vi "PC_Choose_Best_Shot (DONE).vi"(5 "Table Walls Inputs":sgl[](array[numeric]), 6 "Straight/Bounce":bool, 7 "Puck and Players In":T3, 8 "Error In":errorcluster, 10 "Shot Inputs":cluster{"Bounce":dbl[][], "Straight":dbl[][]}, 11 "Image In":T2) -> (0 "Error Out":errorcluster, 1 "Shot Coordinate":T1, 2 "Best Shot Theta":dbl, 3 "Image Out":T2)   [LabVIEW 2017]
uses:
  <vilib>/vision/Image Controls.llb/IMAQ Image.ctl
panel:
  in  "Wall 1 Angle FF":dbl=4.5 format="%#_13g"
  in  "Wall 3 Angle FF":dbl=2.4 format="%#_13g"
  in  "Shot Coordinate Template":T1
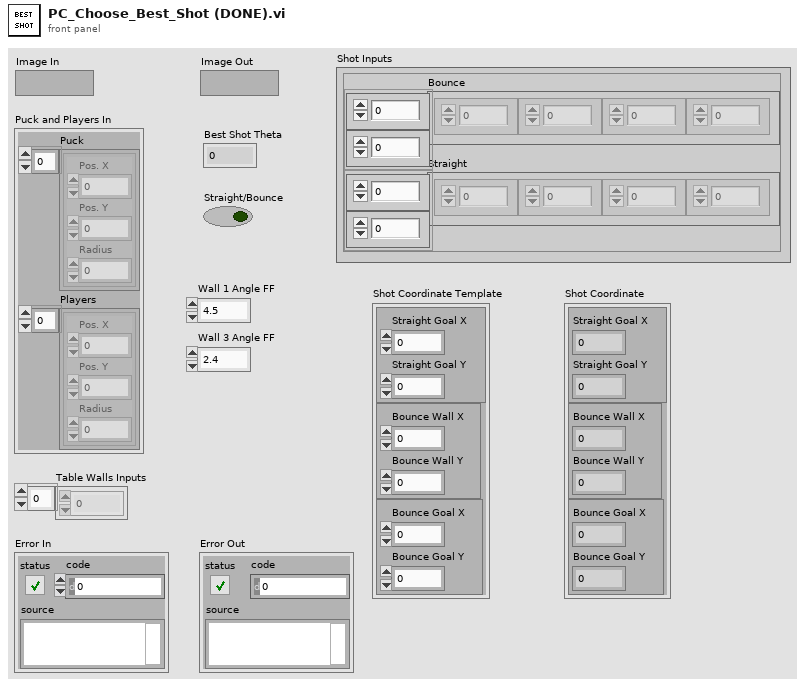
[diagram p1: front panel]
types:
  T1 = cluster{cluster{"Straight Goal X":sgl, "Straight Goal Y":dbl}, cluster{"Bounce Wall X":dbl, "Bounce Wall Y":sgl}, cluster{"Bounce Goal X":sgl, "Bounce Goal Y":dbl}}
  T2 = typedef "IMAQ Image.ctl" = refnum<image>
  T3 = cluster{"Puck":cluster{"Pos. X":i32, "Pos. Y":i32, "Radius":i32}[], "Players":cluster{"Pos. X":i32, "Pos. Y":i32, "Radius":i32}[]}
  T4 = cluster{"Pos. X":i32, "Pos. Y":i32, "Radius":i32}[]
  T5 = cluster{"Pos. X":i32, "Pos. Y":i32, "Radius":i32}
  T6 = cluster{"Numeric Control":sgl, "Numeric Control":dbl}
  T7 = cluster{"Numeric Control":dbl, "Numeric Control":sgl}
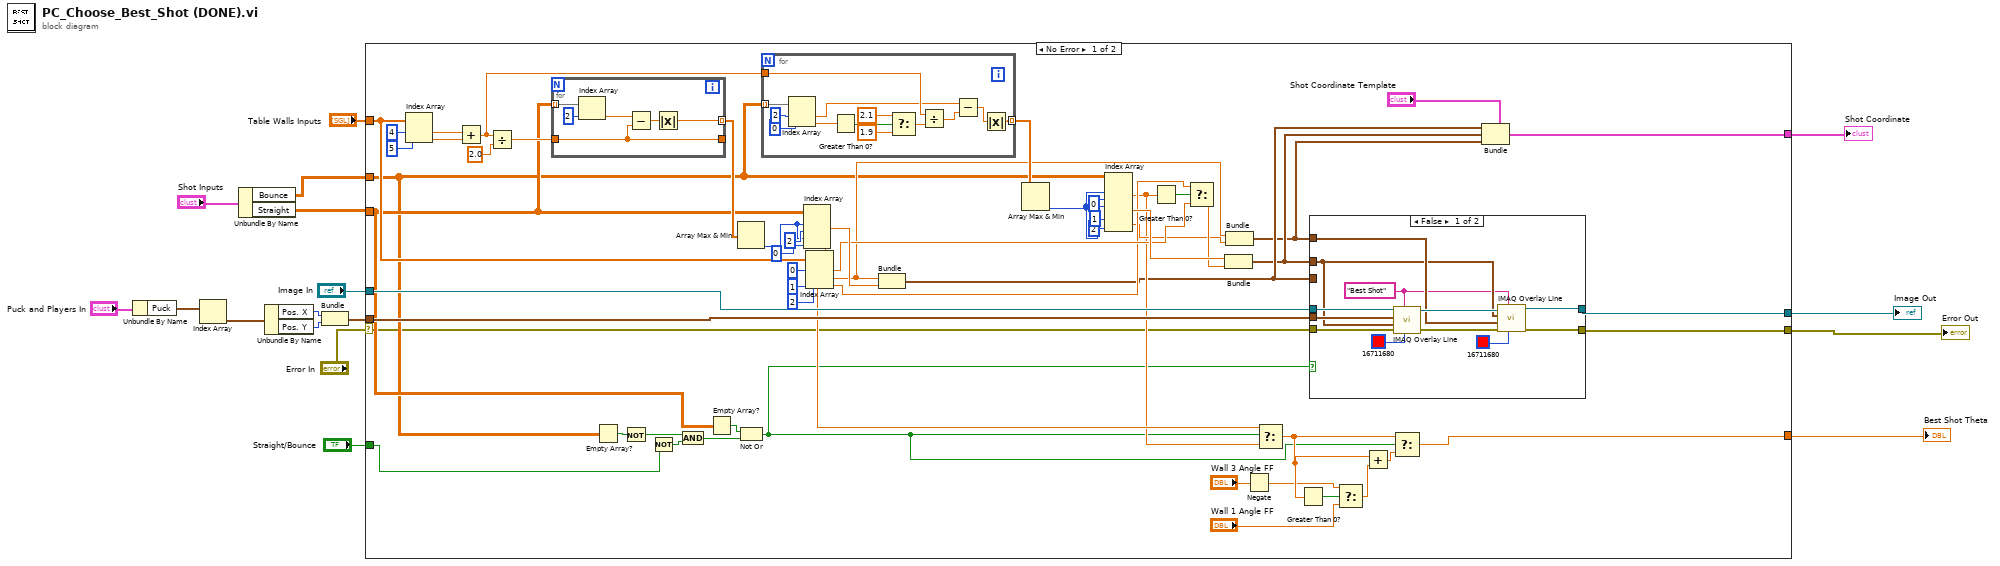
[diagram p0: block diagram]
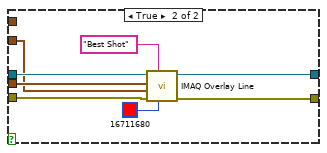
[diagram p2: hidden frame]
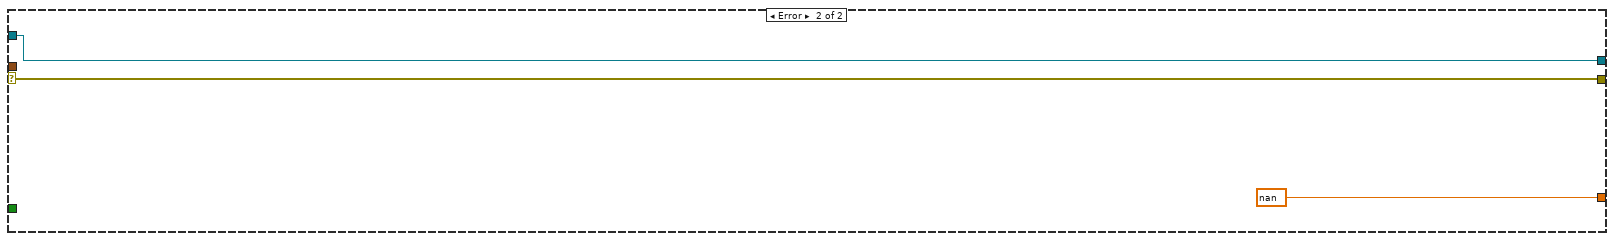
[diagram p3: hidden frame]
diagram:
  n1 = Unbundle By Name("Puck and Players In") -> ("Puck"=w17:T4)
  n2 = Index Array(array=w17) -> (element=w16:T5)  [unwired: 1 in]
  n3 = Unbundle By Name("Shot Inputs") -> ("Bounce"=w3:dbl[][], "Straight"=w2:dbl[][])
  n4 = Unbundle By Name(w16) -> ("Pos. X"=w15:i32, "Pos. Y"=w14:i32)
  n5 = Bundle("Pos. X"=w15, "Pos. Y"=w14) -> (w11:cluster{"Pos. X":i32, "Pos. Y":i32})  [unwired: 1 in]
  n6 = case shown="No Error" "Error In" {
    selector: "Error In" -> [w34 w116]
    tunnel: "Table Walls Inputs" -> [w65 _]
    tunnel: w11 -> [w62 _]
    tunnel: "Image In" -> [w61 w115]
    tunnel: [w60 w116] -> w9
    tunnel: [w59 w115] -> w8
    tunnel: [w27 nan ("Numeric Control")] -> w7
    tunnel: w2 -> [w40 _]
    tunnel: w3 -> [w39 _]
    tunnel: "Straight/Bounce" -> [w28 _]
    tunnel: [w29 _] -> w1
    frame No Error {
      n7 = Index Array(array=w65, index #1=4 ("index"), index #2=5 ("index")) -> (element #1=w72:sgl, element #2=w71:sgl)
      n8 = Add(x=w72, y=w71) -> (x+y=w18:sgl)
      n9 = Divide(x=w18, y=sgl 2.0) -> (x/y=w42:sgl)
      n10 = for {
        tunnel: w40 -> [w113] mode=indexing
        tunnel: w42 -> [w108]
        tunnel: [w109] -> w69 mode=indexing
        tunnel: [w108] -> _
        n11 = Index Array(array=w113, index=2) -> (element=w111:dbl)
        n12 = Subtract(x=w111, y=w108) -> (x-y=w110:dbl)
        n13 = Absolute Value(x=w110) -> (abs(x)=w109:dbl)
      }
      n14 = Empty Array?(array=w39) -> (empty?=w37:bool)
      n15 = Not(x=w37) -> (.not. x?=w36:bool)
      n16 = Not(x=w28) -> (.not. x?=w35:bool)
      n17 = And(x=w36, y=w35) -> (x .and. y?=w41:bool)
      n18 = Empty Array?(array=w40) -> (empty?=w38:bool)
      n19 = Array Max & Min(array=w69) -> (min index (indices)=w46:i32)  [unwired: 3 out]
      n20 = Not Or(1:w41, 2:w38) -> (0:w19:bool)
      n21 = for {
        tunnel: w39 -> [w107] mode=indexing
        tunnel: w18 -> [w98]
        tunnel: [w105] -> w68 mode=indexing
        n22 = Index Array(array=w107, index #1=2 ("index"), index #2=0 ("index")) -> (element #1=w97:dbl, element #2=w103:dbl)
        n23 = Greater Than 0?(x=w103) -> (x > 0?=w102:bool)
        n24 = Select(t=2.1, s=w102, f=1.9) -> (s? t:f=w99:dbl)
        n25 = Divide(x=w98, y=w99) -> (x/y=w96:dbl)
        n26 = Subtract(x=w97, y=w96) -> (x-y=w95:dbl)
        n27 = Absolute Value(x=w95) -> (abs(x)=w105:dbl)
      }
      n28 = Index Array(array=w40, index (row) #1=w46, index (col) #1=2 ("disabled index (col)"), index (row) #2=w46, index (col) #2=0 ("disabled index (col)")) -> (element #1=w63:dbl, element #2=w44:dbl)
      n29 = Index Array(array=w65, index #1=0 ("index"), index #2=1 ("index"), index #3=2 ("index")) -> (element #1=w53:sgl, element #2=w49:sgl, element #3=w50:sgl)
      n30 = Bundle("Numeric Control"=w49, "Numeric Control"=w63) -> (w33:T6)  [unwired: 1 in]
      n31 = Array Max & Min(array=w68) -> (min index (indices)=w47:i32)  [unwired: 3 out]
      n32 = Index Array(array=w39, index (row) #1=w47, index (col) #1=0 ("disabled index (col)"), index (row) #2=w47, index (col) #2=1 ("disabled index (col)"), index (row) #3=w47, index (col) #3=2 ("index (col)")) -> (element #1=w43:dbl, element #2=w56:dbl, element #3=w48:dbl)
      n33 = Greater Than 0?(x=w43) -> (x > 0?=w54:bool)
      n34 = Select(t=w50, s=w54, f=w53) -> (s? t:f=w51:sgl)
      n35 = Bundle("Numeric Control"=w56, "Numeric Control"=w51) -> (w32:T7)  [unwired: 1 in]
      n36 = Bundle("Numeric Control"=w49, "Numeric Control"=w48) -> (w31:T6)  [unwired: 1 in]
      n37 = Negate(x="Wall 3 Angle FF") -> (-x=w22:dbl)
      n38 = Select(t=w44, s=w19, f=w43) -> (s? t:f=w25:dbl)
      n39 = Greater Than 0?(x=w25) -> (x > 0?=w24:bool)
      n40 = case shown="False" w19 {
        tunnel: w34 -> [w84 w93]
        tunnel: w62 -> [w79 w92]
        tunnel: w61 -> [w83 w91]
        tunnel: [w85 w90] -> w60
        tunnel: [w86 w89] -> w59
        tunnel: w33 -> [_ w88]
        tunnel: w32 -> [w76 _]
        tunnel: w31 -> [w77 _]
        frame False {
          w75 = "Best Shot" ("Group")
          n41 = call "IMAQ Overlay Line"("Color"=u32 16711680, "Group"=w75, "error in (no error)"=w84, "End Point"=w76, "Start Point"=w79, "Image"=w83) -> ("error out"=w81:errorcluster, "Image Out"=w80:T2)  [unwired: 4 in]
          n42 = call "IMAQ Overlay Line"("Color"=u32 16711680, "Group"=w75, "error in (no error)"=w81, "End Point"=w77, "Start Point"=w76, "Image"=w80) -> ("error out"=w85:errorcluster, "Image Out"=w86:T2)  [unwired: 4 in]
        }
        frame True {
          n43 = call "IMAQ Overlay Line"("Color"=u32 16711680, "Group"="Best Shot", "error in (no error)"=w93, "End Point"=w88, "Start Point"=w92, "Image"=w91) -> ("error out"=w90:errorcluster, "Image Out"=w89:T2)  [unwired: 4 in]
        }
      }
      n44 = Select(t=w22, s=w24, f="Wall 1 Angle FF") -> (s? t:f=w23:dbl)
      n45 = Add(x=w25, y=w23) -> (x+y=w26:dbl)
      n46 = Select(t=w25, s=w19, f=w26) -> (s? t:f=w27:dbl)
      n47 = Bundle(cluster="Shot Coordinate Template", w33, w32, w31) -> (w29:T1)
    }
    frame Error {
    }
  }
  "Image Out" <- w8
  "Error Out" <- w9
  "Best Shot Theta" <- w7
  "Shot Coordinate" <- w1
